vi "getClickFromSound.vi"() -> ()   [LabVIEW 2011]
uses:
  Kinect softaware needed/Project2 Ni/kinect-1-4/average Y.vi
panel:
  out "click 2":bool
  in  "stop":bool
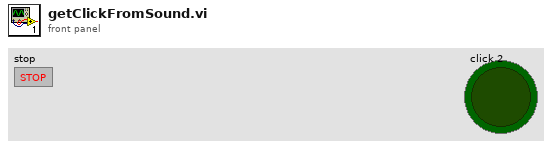
[diagram p1: front panel]
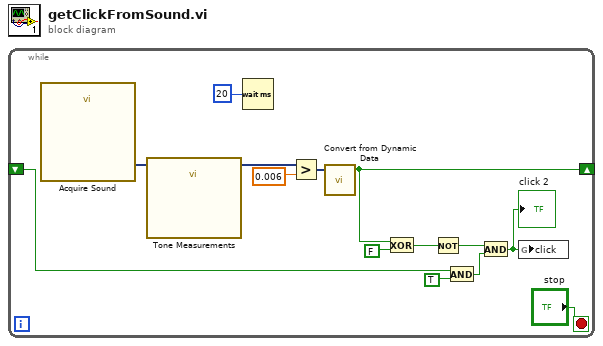
[diagram p0: block diagram]
diagram:
  n1 = while {
    shift-right: [w7] -> _
    shift-left: _ -> [w8]
    stop <- "stop" stop-if-true
    n2 = call "Acquire Sound"() -> ("Data"=w13:dynamicdata)  [unwired: 18 in, 1 out]
    n3 = call "Tone Measurements"("Signals"=w13) -> ("Amplitude"=w12:dynamicdata)  [unwired: 9 in, 1 out]
    n4 = Wait (ms)(milliseconds to wait=u32 20) -> ()  [unwired: 1 out]
    n5 = Greater?(x=w12, y=0.006) -> (0:w10:dynamicdata)
    n6 = call "Convert from Dynamic Data"("Dynamic Data Type"=w10) -> ("Scalar"=w7:bool)  [unwired: 3 in]
    n7 = Exclusive Or(1:FALSE, 2:w7) -> (0:w5:bool)
    n8 = Not(x=w5) -> (.not. x?=w4:bool)
    n9 = And(x=w8, y=TRUE) -> (x .and. y?=w3:bool)
    n10 = And(x=w4, y=w3) -> (x .and. y?=w2:bool)
    "click 2" <- w2
    n11 = global write "average Y.vi" "click"(w2) -> ()
  }
